vi "Resend.vi"(8 "error in (no error)":errorcluster, 11 "BaseDriver in":refnum<class "BaseDriver.lvclass">) -> (0 "error out":errorcluster, 3 "BaseDriver out":refnum<class "BaseDriver.lvclass">)   [LabVIEW 2013, in "BaseDriver.lvclass"]
doc: "Resend the last sent message again"
uses:
  BaseDriver.lvclass
  BaseDriver.lvclass/BaseDriver.ctl
  Reader/BaseReader/BaseReader.lvclass
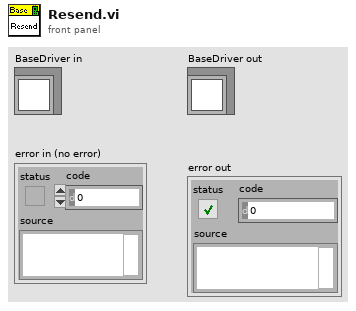
[diagram p1: front panel]
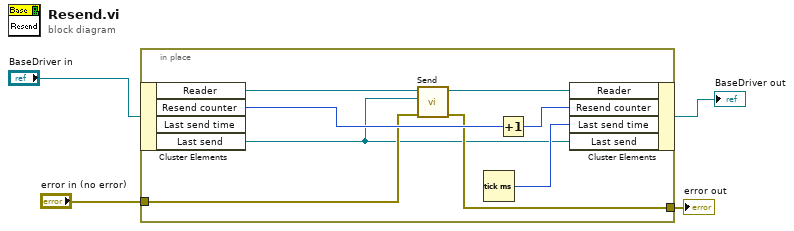
[diagram p0: block diagram]
diagram:
  n1 = in-place "In Place Element Structure" {
    in-place-border: "error in (no error)" -> [w6]
    in-place-border: [w7] -> w2
    n2 = in-place-cluster #1("BaseDriver in") -> ("Reader"=w12:refnum<class "BaseReader.lvclass">, "Resend counter"=w10:i32, "Last send"=w5:refnum<class "BaseMessage.lvclass">)  [unwired: 1 out]
    n3 = call-dynamic "Send.vi"("error in (no error)"=w6, "Message"=w5, "BaseReader in"=w12) -> ("error out"=w7:errorcluster, "BaseReader out"=w11:refnum<class "BaseReader.lvclass">)  [unwired: 6 in, 1 out]
    n4 = Tick Count (ms)() -> (millisecond timer value=w8:u32)
    n5 = Increment(x=w10) -> (x+1=w9:i32)
    n6 = in-place-cluster #1("Reader"=w11, "Resend counter"=w9, "Last send time"=w8, "Last send"=w5) -> (→"BaseDriver out":refnum<class "BaseDriver.lvclass">)
  }
  "error out" <- w2
